vi "unpack DRAM data.vi"(8 "input valid?":bool, 10 "DRAM pack index in":T1, 11 "packer in":T2) -> (0 "output valid?":bool, 1 "Unpacked data":u32, 2 "DRAM pack index out":T1, 3 "packer out":T2)   [LabVIEW 2015]
uses:
  DRAM data index.ctl
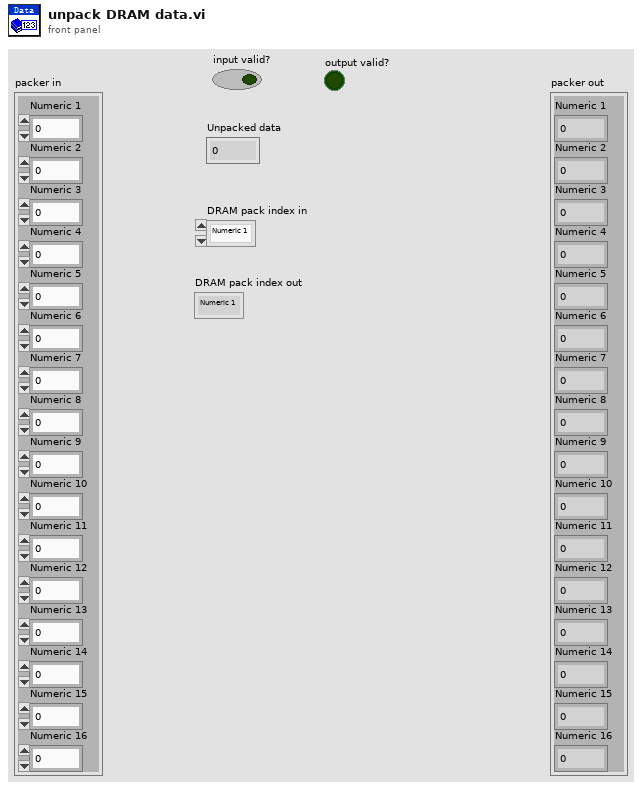
[diagram p1: front panel]
types:
  T1 = typedef "DRAM data index.ctl" = enum16{"Numeric 1", "Numeric 2", "Numeric 3", "Numeric 4", "Numeric 5", "Numeric 6", "Numeric 7", "Numeric 8", "Numeric 9", "Numeric 10", "Numeric 11", "Numeric 12", "Numeric 13", "Numeric 14", "Numeric 15", "Numeric 16"}
  T2 = cluster{"Numeric 1":u32, "Numeric 2":u32, "Numeric 3":u32, "Numeric 4":u32, "Numeric 5":u32, "Numeric 6":u32, "Numeric 7":u32, "Numeric 8":u32, "Numeric 9":u32, "Numeric 10":u32, "Numeric 11":u32, "Numeric 12":u32, "Numeric 13":u32, "Numeric 14":u32, "Numeric 15":u32, "Numeric 16":u32}
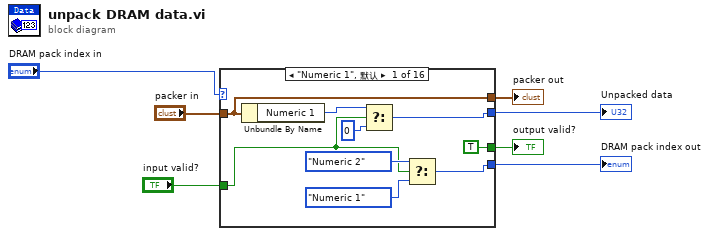
[diagram p0: block diagram]
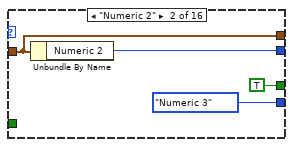
[diagram p2: hidden frame]
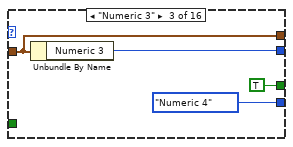
[diagram p3: hidden frame]
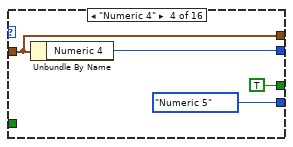
[diagram p4: hidden frame]
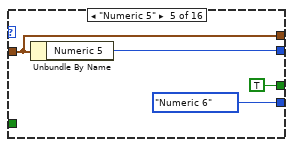
[diagram p5: hidden frame]
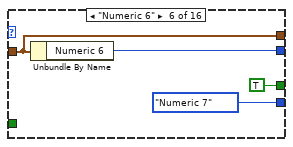
[diagram p6: hidden frame]
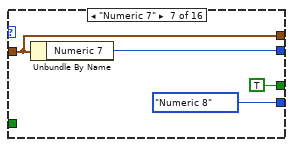
[diagram p7: hidden frame]
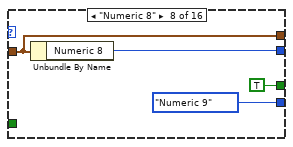
[diagram p8: hidden frame]
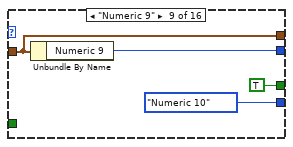
[diagram p9: hidden frame]
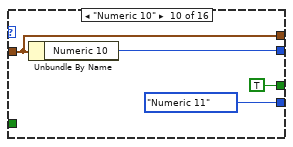
[diagram p10: hidden frame]
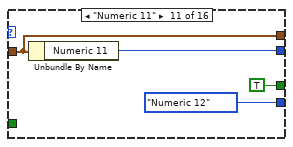
[diagram p11: hidden frame]
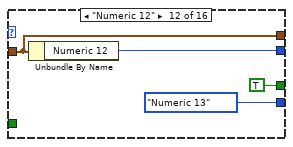
[diagram p12: hidden frame]
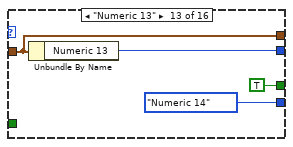
[diagram p13: hidden frame]
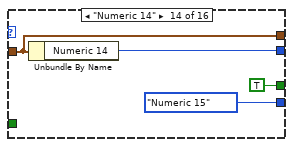
[diagram p14: hidden frame]
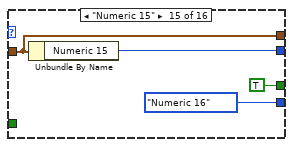
[diagram p15: hidden frame]
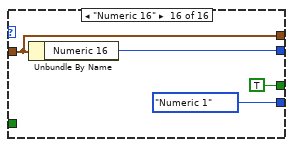
[diagram p16: hidden frame]
diagram:
  n1 = case shown="\"Numeric 1\", 默认" "DRAM pack index in" {
    tunnel: "input valid?" -> [w9 _ _ _ _ _ _ _ _ _ _ _ _ _ _ _]
    tunnel: "packer in" -> [w13 w18 w22 w26 w30 w34 w38 w42 w46 w50 w54 w58 w62 w66 w70 w74]
    tunnel: [w16 DRAM_data_index."Numeric 3" ("Galvo index in") DRAM_data_index."Numeric 4" ("Galvo index in") DRAM_data_index."Numeric 5" ("Galvo index in") DRAM_data_index."Numeric 6" ("Galvo index in") DRAM_data_index."Numeric 7" ("Galvo index in") DRAM_data_index."Numeric 8" ("Galvo index in") DRAM_data_index."Numeric 9" ("Galvo index in") DRAM_data_index."Numeric 10" ("Galvo index in") DRAM_data_index."Numeric 11" ("Galvo index in") DRAM_data_index."Numeric 12" ("Galvo index in") DRAM_data_index."Numeric 13" ("Galvo index in") DRAM_data_index."Numeric 14" ("Galvo index in") DRAM_data_index."Numeric 15" ("Galvo index in") DRAM_data_index."Numeric 16" ("Galvo index in") DRAM_data_index."Numeric 1" ("Galvo index in")] -> w1
    tunnel: [TRUE TRUE TRUE TRUE TRUE TRUE TRUE TRUE TRUE TRUE TRUE TRUE TRUE TRUE TRUE TRUE] -> w5
    tunnel: [w10 w19 w23 w27 w31 w35 w39 w43 w47 w51 w55 w59 w63 w67 w71 w75] -> w4
    tunnel: [w13 w18 w22 w26 w30 w34 w38 w42 w46 w50 w54 w58 w62 w66 w70 w74] -> w3
    frame "Numeric 1", Default {
      n2 = Unbundle By Name(w13) -> ("Numeric 1"=w12:u32)
      n3 = Select(t=w12, s=w9, f=u32 0) -> (s? t:f=w10:u32)
      n4 = Select(t=DRAM_data_index."Numeric 2" ("Galvo index in"), s=w9, f=DRAM_data_index."Numeric 1" ("Galvo index in")) -> (s? t:f=w16:T1)
    }
    frame "Numeric 2" {
      n5 = Unbundle By Name(w18) -> ("Numeric 2"=w19:u32)
    }
    frame "Numeric 3" {
      n6 = Unbundle By Name(w22) -> ("Numeric 3"=w23:u32)
    }
    frame "Numeric 4" {
      n7 = Unbundle By Name(w26) -> ("Numeric 4"=w27:u32)
    }
    frame "Numeric 5" {
      n8 = Unbundle By Name(w30) -> ("Numeric 5"=w31:u32)
    }
    frame "Numeric 6" {
      n9 = Unbundle By Name(w34) -> ("Numeric 6"=w35:u32)
    }
    frame "Numeric 7" {
      n10 = Unbundle By Name(w38) -> ("Numeric 7"=w39:u32)
    }
    frame "Numeric 8" {
      n11 = Unbundle By Name(w42) -> ("Numeric 8"=w43:u32)
    }
    frame "Numeric 9" {
      n12 = Unbundle By Name(w46) -> ("Numeric 9"=w47:u32)
    }
    frame "Numeric 10" {
      n13 = Unbundle By Name(w50) -> ("Numeric 10"=w51:u32)
    }
    frame "Numeric 11" {
      n14 = Unbundle By Name(w54) -> ("Numeric 11"=w55:u32)
    }
    frame "Numeric 12" {
      n15 = Unbundle By Name(w58) -> ("Numeric 12"=w59:u32)
    }
    frame "Numeric 13" {
      n16 = Unbundle By Name(w62) -> ("Numeric 13"=w63:u32)
    }
    frame "Numeric 14" {
      n17 = Unbundle By Name(w66) -> ("Numeric 14"=w67:u32)
    }
    frame "Numeric 15" {
      n18 = Unbundle By Name(w70) -> ("Numeric 15"=w71:u32)
    }
    frame "Numeric 16" {
      n19 = Unbundle By Name(w74) -> ("Numeric 16"=w75:u32)
    }
  }
  "packer out" <- w3
  "output valid?" <- w5
  "Unpacked data" <- w4
  "DRAM pack index out" <- w1
